vi "QPSK Demodulation (SubVI).vi"(11 "pulse shaping filter (none)":T2(ring)) -> (1 "PSK system parameters":T1 {"PSK type" items=["normal", "shifted", "offset"]; "symbol map" format="%.3f"}, 2 "matched filter coefficients":dbl[](array[numeric]), 3 "QPSK synchronization parameters":T3, 4 "output bit stream":i8[](array[numeric]))   [LabVIEW 2026]
uses:
  <vilib>/addons/Modulation/Digital/General/MT Generate Bits (Galois, PN Order).vi
  <vilib>/addons/Modulation/Digital/Support/Common/Validators/mod_Generate Bits Validate.vi
  <vilib>/addons/Modulation/Analog/support/mod_Set Error Source.vi
  <vilib>/addons/Modulation/Digital/General/subVIs/mod_Generate Bits PN Sequence.vi
  <vilib>/addons/Modulation/Digital/General/MT Generate PSK System Parameters(M).vi
  <vilib>/addons/Modulation/Digital/General/MT Generate PSK Synchronization Parameters (bit array).vi
  <vilib>/addons/Modulation/Digital/Support/Common/Validators/mod_Generate Filter Coefficients Validate.vi
  <vilib>/addons/Modulation/Digital/General/subVIs/mod_Generate Filter Coefficients.vi
  <vilib>/addons/Modulation/niDMT.lvlib
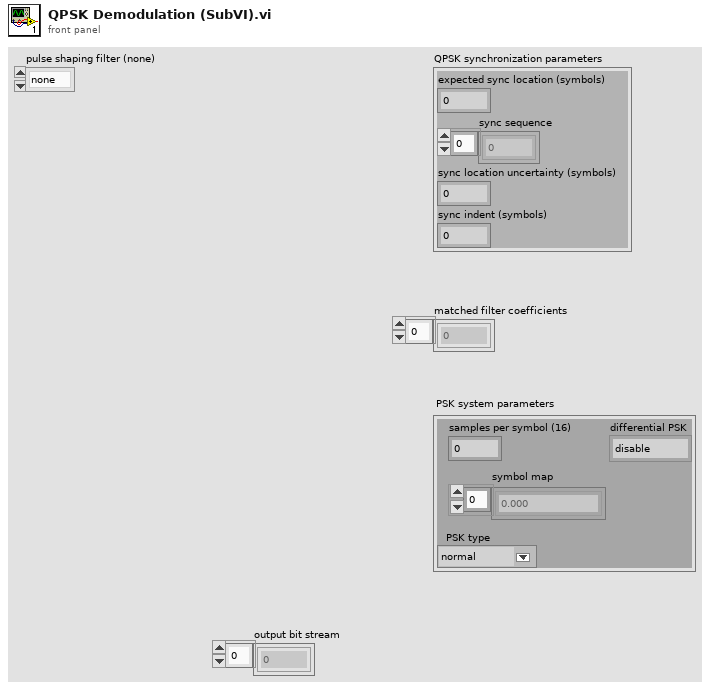
[diagram p1: front panel]
types:
  T1 = cluster{"samples per symbol (16)":i32, "symbol map":cdb[], "differential PSK":enum16{"disable", "enable"}, "PSK type":u16}
  T2 = enum16{"none", "Raised Cosine", "Root Raised Cos", "Gaussian"}
  T3 = cluster{"expected sync location (symbols)":i32, "sync sequence":cdb[], "sync location uncertainty (symbols)":i32, "sync indent (symbols)":i32}
  T4 = enum16{"FSK", "PSK", "QAM", "MSK", "PAM", "ASK", "CPM"}
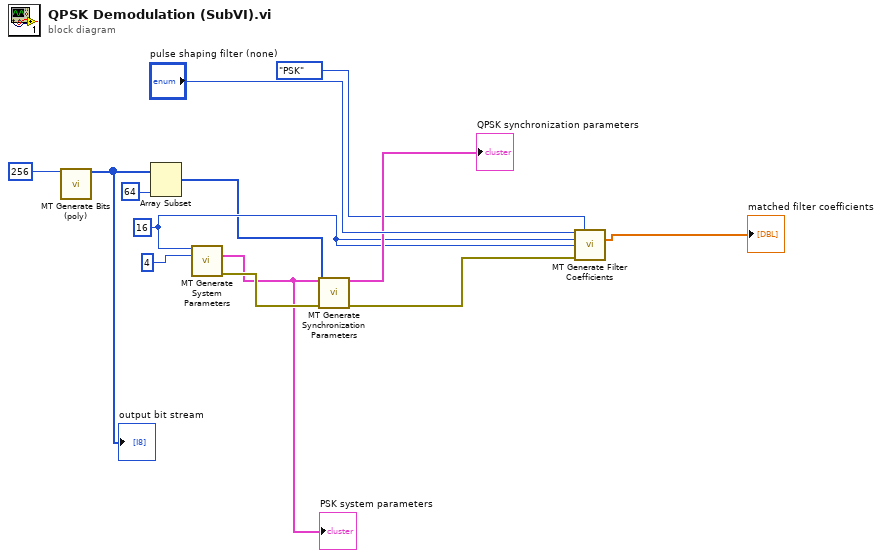
[diagram p0: block diagram]
diagram:
  w3 = 16 ("samples per symbol (16)")
  n1 = call-poly <vilib>:"MT Generate Bits (poly).vi"("total bits (128)"=256) -> ("output bit stream"=w1:i8[])  [unwired: 12 in, 2 out]
  "output bit stream" <- w1
  n2 = Array Subset(array=w1, length=64) -> (w2:i8[])  [unwired: 1 in]
  n3 = call-poly <vilib>:"MT Generate System Parameters.vi"("samples per symbol (16)"=w3, "M-PSK (4)"=4) -> ("PSK system parameters"=w9:T1, "error out"=w10:errorcluster)  [unwired: 11 in, 1 out]
  "PSK system parameters" <- w9
  n4 = call-poly <vilib>:"MT Generate Synchronization Parameters.vi"("PSK system parameters"=w9, "sync bits"=w2, "error in (no error)"=w10) -> ("PSK synchronization parameters"=→"QPSK synchronization parameters":T3, "error out"=w11:errorcluster)  [unwired: 11 in]
  n5 = call <vilib>:"MT Generate Filter Coefficients.vi"("pulse shaping filter (none)"="pulse shaping filter (none)", "modulation type"=T4."PSK", "pulse shaping samples per symbol (16)"=w3, "matched samples per symbol (16)"=w3, "error in (no error)"=w11) -> ("matched filter coefficients"=→"matched filter coefficients":dbl[])  [unwired: 8 in, 2 out]
